vi "Channels.vi"() -> (3 "Channels to Create":T1[](array[typedef]) {"Custom Config Data" format="%x"})   [LabVIEW 2021, in "CIFTemplatePluginCommon.lvlib"]
uses:
  CIFTemplatePluginCommon.lvlib
  Channels/ChannelRegistrar/typedef/Registered Channel Types.ctl
  Channels/ChannelRegistrar/ChannelRegistrar.lvlib
  Channels/CIFChannels/Typedef/Direction.ctl
  Channels/CIFChannels/CIFChannels.lvclass
  Channels/ChannelRegistrar/typedef/Channel Definition.ctl
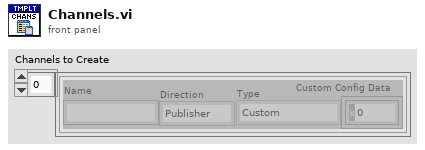
[diagram p1: front panel]
types:
  T1 = typedef "ChannelRegistrar.lvlib/Channel Definition.ctl" = cluster{"Name":string, "Direction":T2, "Type":T3, "Custom Config Data":u8[]}
  T2 = typedef "CIFChannels.lvclass/Direction.ctl" = enum16{"Publisher", "Subscriber"}
  T3 = typedef "ChannelRegistrar.lvlib/Registered Channel Types.ctl" = enum16{"Custom", "CIFTag_Double", "CIFTag_I64", "CIFTag_U64", "CIFFifoCAN"}
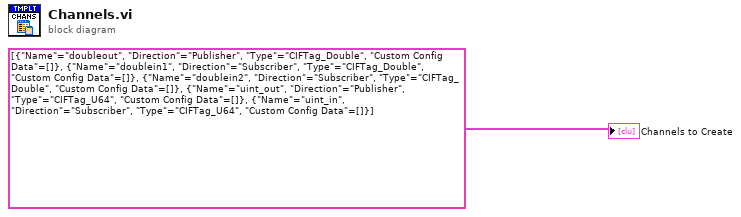
[diagram p0: block diagram]
diagram:
  "Channels to Create" <- T1[] [{"Name"="doubleout", "Direction"=enum."Publisher", "Type"=enum."CIFTag_Double", "Custom Config Data"=[]}, {"Name"="doublein1", "Direction"=enum."Subscriber", "Type"=enum."CIFTag_Double", "Custom Config Data"=[]}, {"Name"="doublein2", "Direction"=enum."Subscriber", "Type"=enum."CIFTag_Double", "Custom Config Data"=[]}, {"Name"="uint_out", "Direction"=enum."Publisher", "Type"=enum."CIFTag_U64", "Custom Config Data"=[]}, {"Name"="uint_in", "Direction"=enum."Subscriber", "Type"=enum."CIFTag_U64", "Custom Config Data"=[]}] ("Channels to Create in")
